vi "Update Shot Table.vi"(1 "Sort by AVG":bool, 2 "Site":string="ICE1", 3 "shotsArr":T1 {"Frag Rod" format="%.1f"; "UncorrectedAvgVel_PB" format="%.1f"; "UncorrectedRed_PB" format="%.1f"; "strikeVel_PB" format="%.1f"; "velLoss_PB" format="%.1f"; "avgVel_PB" format="%.1f"; "Redundant_Velocity" format="%.1f"; "Energy Loss (J)" format="%.3e"; "Projectile Mass" min=0 step=1 format="%.4f"; "Corrected residual" format="%.2f"; "Uncorrected Residual" format="%.1f"; "Corrected Impact" format="%.2f"; "Uncorrected Impact" format="%.1f"; "Shot Angle" max=90 step=1; "SHOT STATUS" items=["Partial", "Complete"]; "IMPACT VELOCITY" min=0 max=10000 step=0.1 format="%.1f"; "Barrel Temperature" format="%.1f"; "Powder Loading" format="%.4f"; "RESIDUAL  VELOCITY" min=0 max=10000 step=0.1 format="%.1f"}) -> (0 "shotTable OUT":string[][](array[string]))   [LabVIEW 2015]
uses:
  shotsArr.ctl
  Shot Record.ctl
panel:
  # "Chrono#1"
  # "Chrono#2"
  # "Average"
  # "Vel Loss"
  # "Strike Vel"
  # "Residual"
  # "Status"
  # "Depth"
  # "Diameter"
  # "Loading"
  # "Description"
  # "Order"
  # "Chrono#1"
  # "Chrono#2"
  # "Strike Vel"
  # "Status"
  # "Depth"
  # "Loading"
  # "Description"
  # "SPR"
  # "Order"
  # "Chrono#1"
  # "Chrono#2"
  # "Strike Vel"
  # "Status"
  # "Depth"
  # "Loading"
  # "Description"
  # "BRZ"
  # "Order"
  # "Corrected"
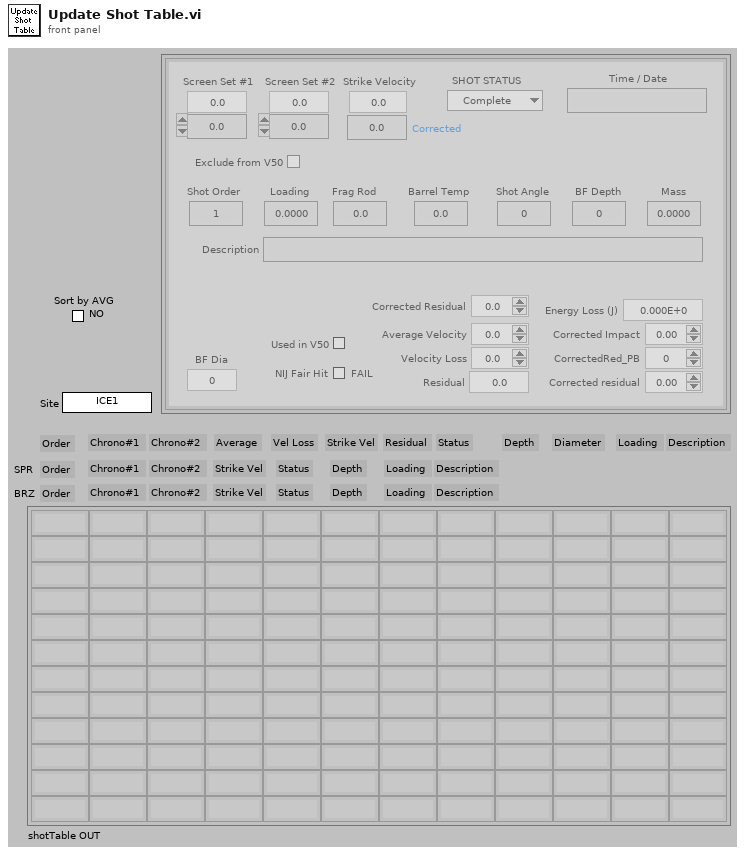
[diagram p1: front panel]
types:
  T1 = typedef "shotsArr.ctl" = T2[]
  T2 = typedef "Shot Record.ctl" = cluster{"Uncorrected Impact":sgl, "Uncorrected Residual":sgl, "avgVel_PB":sgl, "IMPACT VELOCITY":sgl, "RESIDUAL  VELOCITY ":sgl, "Shot Description":string, "Powder Loading ":sgl, "Barrel Temperature":sgl, "TIME / DATE":string, "shot order":i32, "SHOT STATUS":u16, "Shot Angle":u16, "Corrected Impact":sgl, "Corrected residual":sgl, "Projectile Mass":sgl, "usedv50":bool, "Energy Loss (J)":sgl, "BackFace\nDepth":sgl, "BackFace\nDiameter":sgl, "Redundant_Velocity":sgl, "velLoss_PB":sgl, "strikeVel_PB":sgl, "UncorrectedRed_PB":sgl, "CorrectedRed_PB":sgl, "UncorrectedAvgVel_PB":sgl, "V50userExcl":bool, "Frag Rod":sgl, "fairHit":bool}
  T3 = cluster{"[0]":string, "[1]":string, "[2]":string, "[3]":string, "[4]":string, "[5]":string, "[6]":string, "[7]":string, "[8]":string, "[9]":string, "[10]":string, "[11]":string}[]
  T4 = cluster{"[0]":string, "[1]":string, "[2]":string, "[3]":string, "[4]":string, "[5]":string, "[6]":string, "[7]":string, "[8]":string, "[9]":string, "[10]":string, "[11]":string}
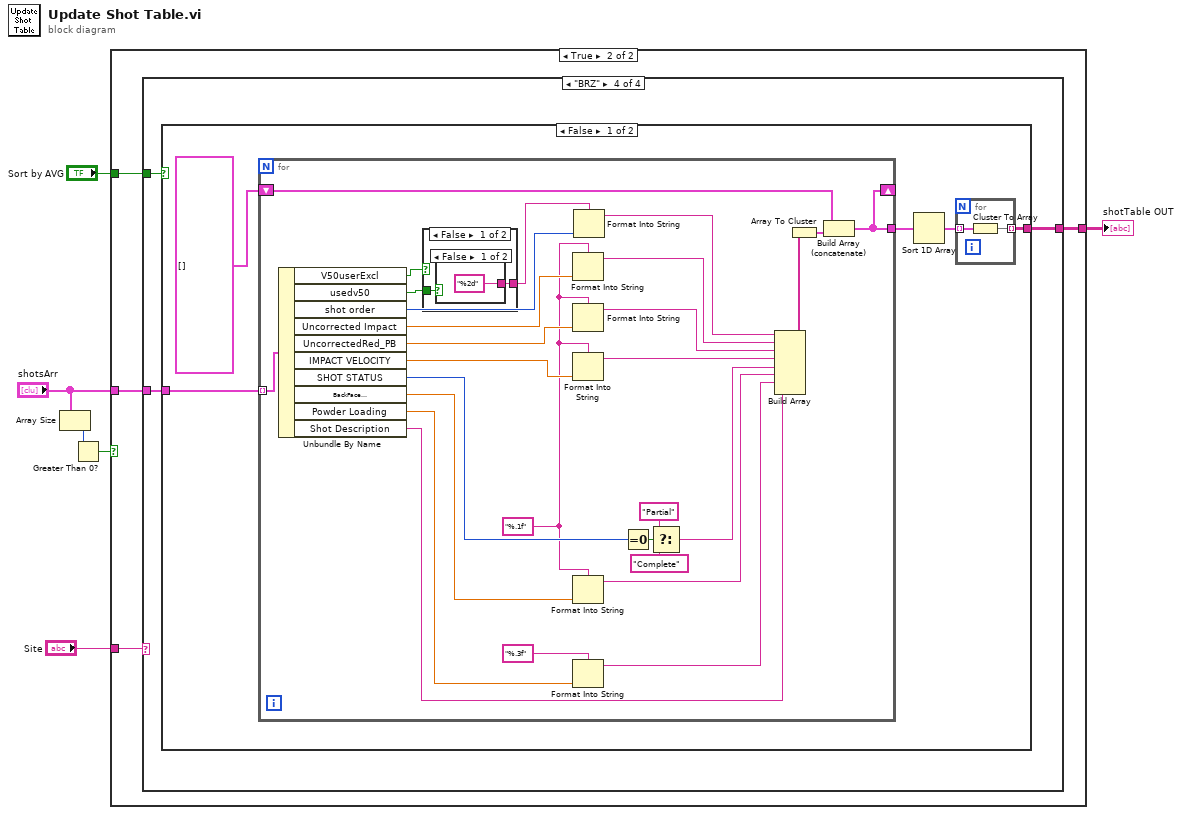
[diagram p0: block diagram]
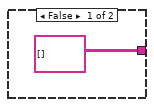
[diagram p2: hidden frame]
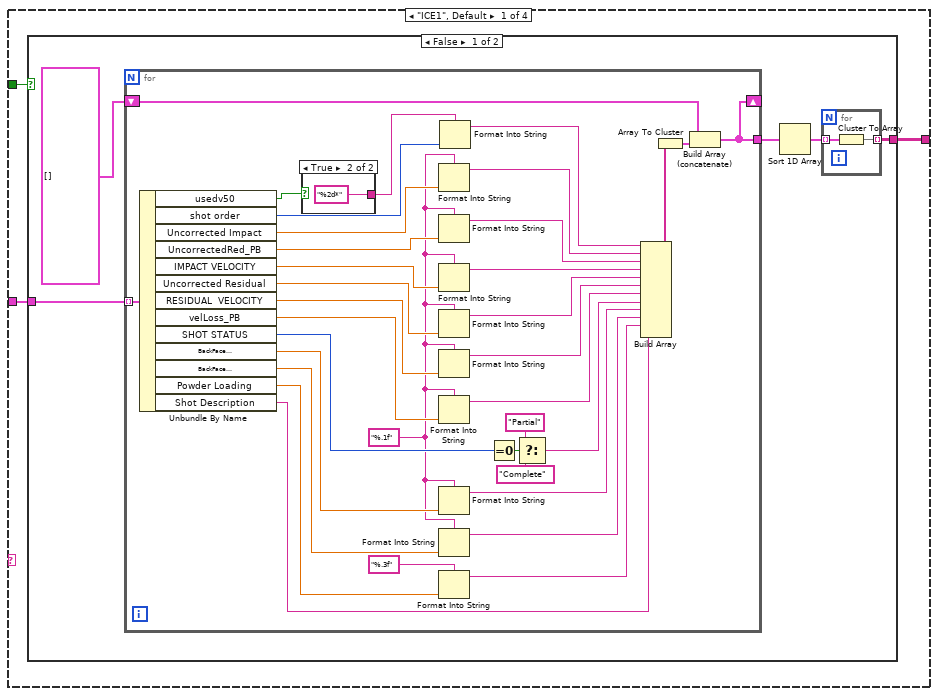
[diagram p3: hidden frame]
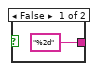
[diagram p4: hidden frame]
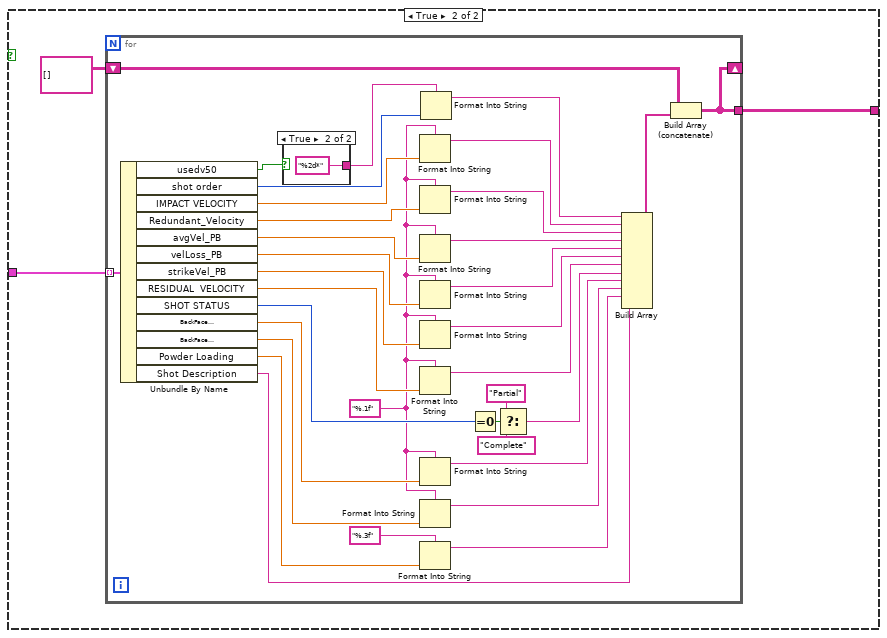
[diagram p5: hidden frame]
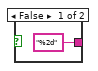
[diagram p6: hidden frame]
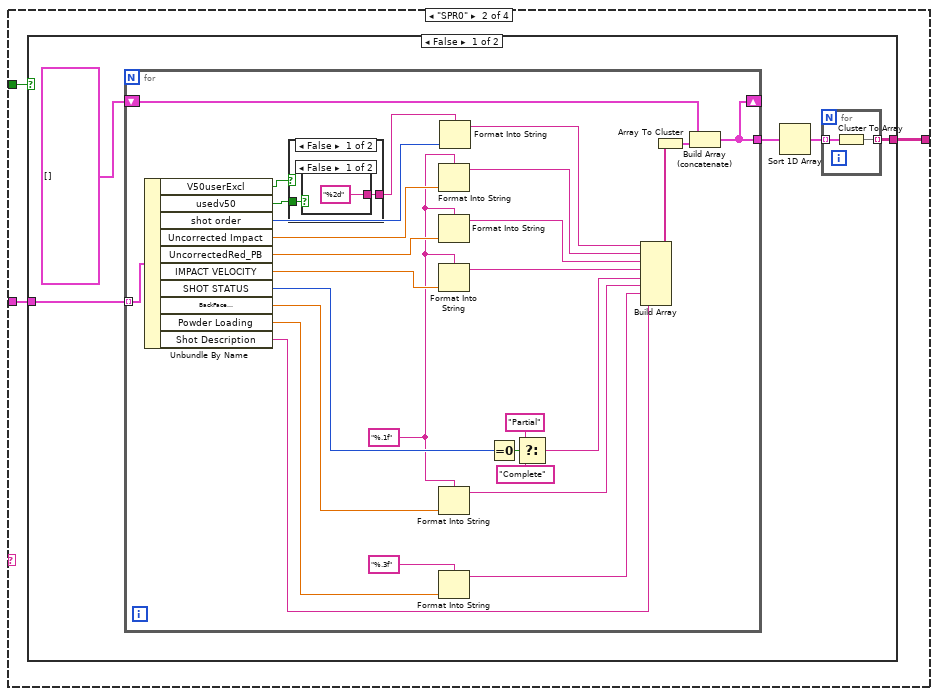
[diagram p7: hidden frame]
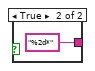
[diagram p8: hidden frame]
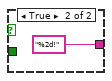
[diagram p9: hidden frame]
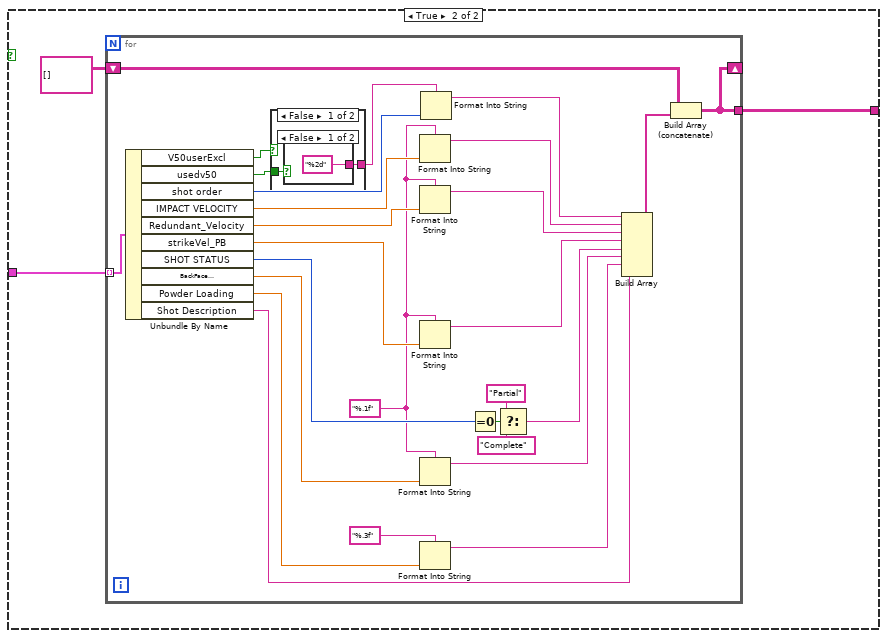
[diagram p10: hidden frame]
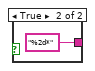
[diagram p11: hidden frame]
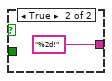
[diagram p12: hidden frame]
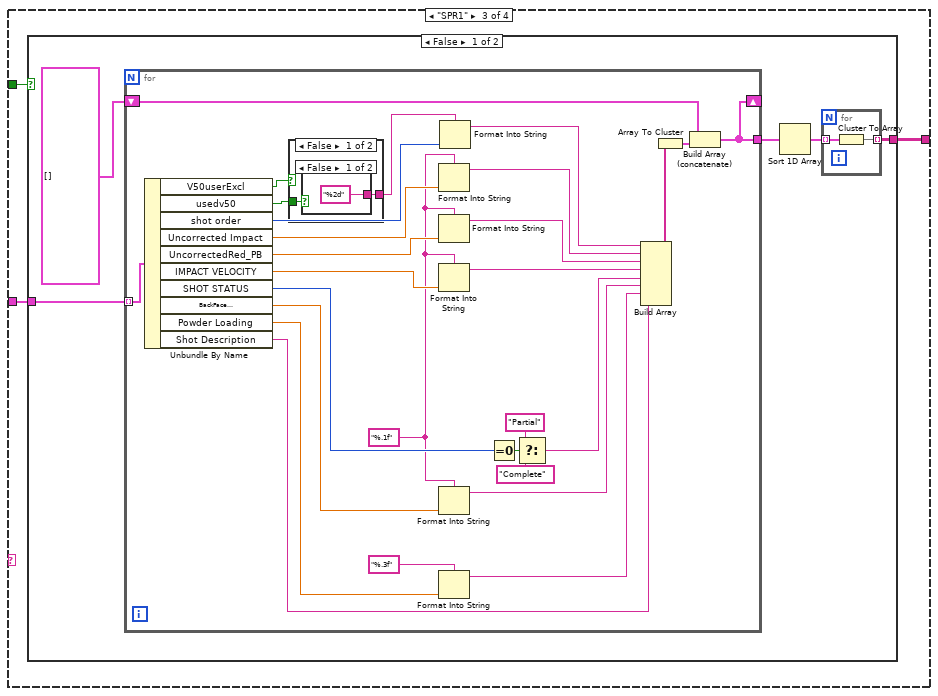
[diagram p13: hidden frame]
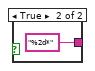
[diagram p14: hidden frame]
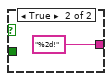
[diagram p15: hidden frame]
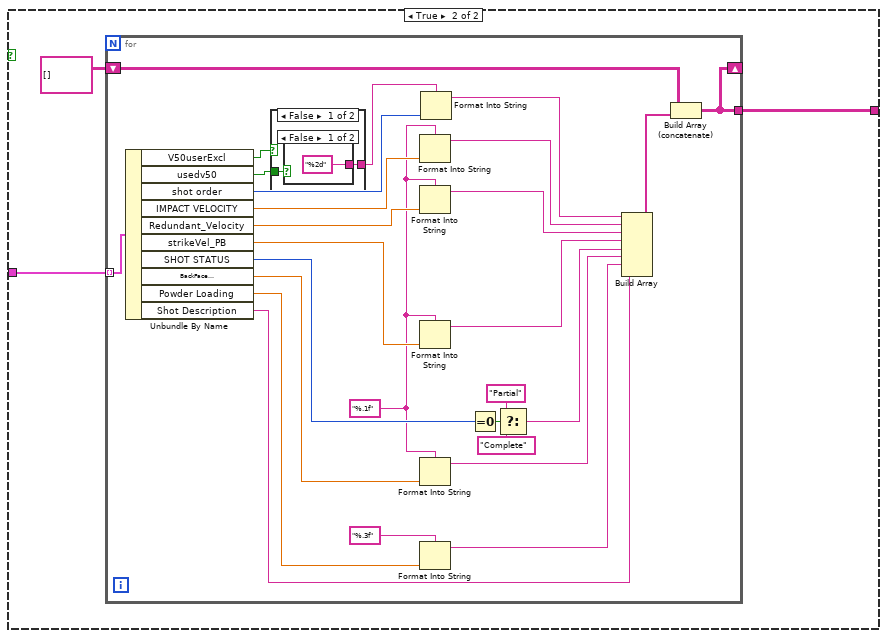
[diagram p16: hidden frame]
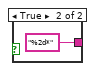
[diagram p17: hidden frame]
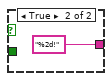
[diagram p18: hidden frame]
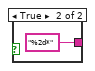
[diagram p19: hidden frame]
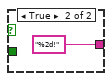
[diagram p20: hidden frame]
diagram:
  n1 = Array Size(array="shotsArr") -> (size(s)=w6:i32)
  n2 = Greater Than 0?(x=w6) -> (x > 0?=w4:bool)
  n3 = case shown="True" w4 {
    tunnel: "shotsArr" -> [_ w11]
    tunnel: [string[][] [] w10] -> w5
    tunnel: "Sort by AVG" -> [_ w9]
    tunnel: "Site" -> [_ w8]
    frame False {
    }
    frame True {
      n4 = case shown="\"BRZ\"" w8 {
        tunnel: w11 -> [w14 w100 w178 w256]
        tunnel: [w13 w99 w177 w255] -> w10
        tunnel: w9 -> [w12 w98 w176 w254]
        frame "ICE1", Default {
          n5 = case shown="False" w12 {
            tunnel: w14 -> [w19 w60]
            tunnel: [w17 w59] -> w13
            frame False {
              n6 = for {
                tunnel: w19 -> [w44] mode=indexing
                shift-right: [w52] -> _
                shift-left: T3 [] -> [w56]
                tunnel: [w52] -> w18
                w23 = "%.1f" ("Format String")
                n7 = Unbundle By Name(w44) -> ("usedv50"=w43:bool, "shot order"=w42:i32, "Uncorrected Impact"=w41:sgl, "UncorrectedRed_PB"=w40:sgl, "IMPACT VELOCITY"=w39:sgl, "Uncorrected Residual"=w38:sgl, "RESIDUAL  VELOCITY"=w37:sgl, "velLoss_PB"=w31:sgl, "SHOT STATUS"=w27:u16, "BackFace\nDepth"=w36:sgl, "BackFace\nDiameter"=w35:sgl, "Powder Loading"=w34:sgl, "Shot Description"=w33:string)
                n8 = case shown="True" w43 {
                  tunnel: ["%2d" "%2d*"] -> w51
                  frame False {
                  }
                  frame True {
                  }
                }
                n9 = Format Into String(format string=w23, w41) -> (resulting string=w53:string)  [unwired: 2 in, 1 out]
                n10 = Format Into String(format string=w23, w40) -> (resulting string=w54:string)  [unwired: 2 in, 1 out]
                n11 = Format Into String(format string=w23, w39) -> (resulting string=w32:string)  [unwired: 2 in, 1 out]
                n12 = Format Into String(format string=w23, w38) -> (resulting string=w49:string)  [unwired: 2 in, 1 out]
                n13 = Format Into String(format string=w23, w37) -> (resulting string=w48:string)  [unwired: 2 in, 1 out]
                n14 = Format Into String(format string=w23, w31) -> (resulting string=w25:string)  [unwired: 2 in, 1 out]
                n15 = Format Into String(format string=w23, w36) -> (resulting string=w47:string)  [unwired: 2 in, 1 out]
                n16 = Format Into String(format string=w23, w35) -> (resulting string=w46:string)  [unwired: 2 in, 1 out]
                n17 = Format Into String(format string="%.3f" ("Format String"), w34) -> (resulting string=w45:string)  [unwired: 2 in, 1 out]
                n18 = Format Into String(format string=w51, w42) -> (resulting string=w50:string)  [unwired: 2 in, 1 out]
                n19 = Equal To 0?(x=w27) -> (x = 0?=w28:bool)
                n20 = Select(t="Partial", s=w28, f="Complete") -> (s? t:f=w26:string)
                n21 = Build Array(w50, w53, w54, w32, w49, w48, w25, w26, w47, w46, w45, w33) -> (w55:string[])
                n22 = Array To Cluster(array=w55) -> (cluster=w22:T4)
                n23 = Build Array (concatenate)(w56, w22) -> (w52:T3)
              }
              n24 = Sort 1D Array(array=w18) -> (sorted array=w15:T3)
              n25 = for {
                tunnel: w15 -> [w21] mode=indexing
                tunnel: [w20] -> w17 mode=indexing
                n26 = Cluster To Array(cluster=w21) -> (array=w20:string[])
              }
            }
            frame True {
              n27 = for {
                tunnel: w60 -> [w84] mode=indexing
                shift-right: [w92] -> _
                shift-left: string[][] [] -> [w95]
                tunnel: [w92] -> w59
                w63 = "%.1f" ("Format String")
                n28 = Unbundle By Name(w84) -> ("usedv50"=w83:bool, "shot order"=w82:i32, "IMPACT VELOCITY"=w81:sgl, "Redundant_Velocity"=w80:sgl, "avgVel_PB"=w79:sgl, "velLoss_PB"=w78:sgl, "strikeVel_PB"=w77:sgl, "RESIDUAL  VELOCITY"=w71:sgl, "SHOT STATUS"=w67:u16, "BackFace\nDepth"=w76:sgl, "BackFace\nDiameter"=w75:sgl, "Powder Loading"=w74:sgl, "Shot Description"=w73:string)
                n29 = case shown="True" w83 {
                  tunnel: ["%2d" "%2d*"] -> w91
                  frame False {
                  }
                  frame True {
                  }
                }
                n30 = Format Into String(format string=w63, w81) -> (resulting string=w93:string)  [unwired: 2 in, 1 out]
                n31 = Format Into String(format string=w63, w80) -> (resulting string=w94:string)  [unwired: 2 in, 1 out]
                n32 = Format Into String(format string=w63, w79) -> (resulting string=w72:string)  [unwired: 2 in, 1 out]
                n33 = Format Into String(format string=w63, w78) -> (resulting string=w89:string)  [unwired: 2 in, 1 out]
                n34 = Format Into String(format string=w63, w77) -> (resulting string=w88:string)  [unwired: 2 in, 1 out]
                n35 = Format Into String(format string=w63, w71) -> (resulting string=w65:string)  [unwired: 2 in, 1 out]
                n36 = Format Into String(format string=w63, w76) -> (resulting string=w87:string)  [unwired: 2 in, 1 out]
                n37 = Format Into String(format string=w63, w75) -> (resulting string=w86:string)  [unwired: 2 in, 1 out]
                n38 = Format Into String(format string="%.3f" ("Format String"), w74) -> (resulting string=w85:string)  [unwired: 2 in, 1 out]
                n39 = Format Into String(format string=w91, w82) -> (resulting string=w90:string)  [unwired: 2 in, 1 out]
                n40 = Equal To 0?(x=w67) -> (x = 0?=w68:bool)
                n41 = Select(t="Partial", s=w68, f="Complete") -> (s? t:f=w66:string)
                n42 = Build Array(w90, w93, w94, w72, w89, w88, w65, w66, w87, w86, w85, w73) -> (w62:string[])
                n43 = Build Array (concatenate)(w95, w62) -> (w92:string[][])
              }
            }
          }
        }
        frame "SPR0" {
          n44 = case shown="False" w98 {
            tunnel: w100 -> [w105 w142]
            tunnel: [w103 w141] -> w99
            frame False {
              n45 = for {
                tunnel: w105 -> [w126] mode=indexing
                shift-right: [w131] -> _
                shift-left: T3 [] -> [w135]
                tunnel: [w131] -> w104
                w110 = "%.1f" ("Format String")
                n46 = Unbundle By Name(w126) -> ("V50userExcl"=w108:bool, "usedv50"=w125:bool, "shot order"=w124:i32, "Uncorrected Impact"=w123:sgl, "UncorrectedRed_PB"=w122:sgl, "IMPACT VELOCITY"=w121:sgl, "SHOT STATUS"=w113:u16, "BackFace\nDepth"=w120:sgl, "Powder Loading"=w119:sgl, "Shot Description"=w118:string)
                n47 = case shown="False" w108 {
                  tunnel: [w137 "%2d!"] -> w130
                  tunnel: w125 -> [w136 _]
                  frame False {
                    n48 = case shown="False" w136 {
                      tunnel: ["%2d" "%2d*"] -> w137
                      frame False {
                      }
                      frame True {
                      }
                    }
                  }
                  frame True {
                  }
                }
                n49 = Format Into String(format string=w110, w123) -> (resulting string=w132:string)  [unwired: 2 in, 1 out]
                n50 = Format Into String(format string=w110, w122) -> (resulting string=w133:string)  [unwired: 2 in, 1 out]
                n51 = Format Into String(format string=w110, w121) -> (resulting string=w117:string)  [unwired: 2 in, 1 out]
                n52 = Format Into String(format string=w110, w120) -> (resulting string=w128:string)  [unwired: 2 in, 1 out]
                n53 = Format Into String(format string="%.3f" ("Format String"), w119) -> (resulting string=w127:string)  [unwired: 2 in, 1 out]
                n54 = Format Into String(format string=w130, w124) -> (resulting string=w129:string)  [unwired: 2 in, 1 out]
                n55 = Equal To 0?(x=w113) -> (x = 0?=w114:bool)
                n56 = Select(t="Partial", s=w114, f="Complete") -> (s? t:f=w112:string)
                n57 = Build Array(w129, w132, w133, w117, w112, w128, w127, w118) -> (w134:string[])
                n58 = Array To Cluster(array=w134) -> (cluster=w109:T4)
                n59 = Build Array (concatenate)(w135, w109) -> (w131:T3)
              }
              n60 = Sort 1D Array(array=w104) -> (sorted array=w101:T3)
              n61 = for {
                tunnel: w101 -> [w107] mode=indexing
                tunnel: [w106] -> w103 mode=indexing
                n62 = Cluster To Array(cluster=w107) -> (array=w106:string[])
              }
            }
            frame True {
              n63 = for {
                tunnel: w142 -> [w162] mode=indexing
                shift-right: [w167] -> _
                shift-left: string[][] [] -> [w170]
                tunnel: [w167] -> w141
                w148 = "%.1f" ("Format String")
                n64 = Unbundle By Name(w162) -> ("V50userExcl"=w145:bool, "usedv50"=w146:bool, "shot order"=w161:i32, "IMPACT VELOCITY"=w160:sgl, "Redundant_Velocity"=w159:sgl, "strikeVel_PB"=w158:sgl, "SHOT STATUS"=w151:u16, "BackFace\nDepth"=w157:sgl, "Powder Loading"=w156:sgl, "Shot Description"=w155:string)
                n65 = case shown="False" w145 {
                  tunnel: [w172 "%2d!"] -> w144
                  tunnel: w146 -> [w171 _]
                  frame False {
                    n66 = case shown="False" w171 {
                      tunnel: ["%2d" "%2d*"] -> w172
                      frame False {
                      }
                      frame True {
                      }
                    }
                  }
                  frame True {
                  }
                }
                n67 = Format Into String(format string=w148, w160) -> (resulting string=w168:string)  [unwired: 2 in, 1 out]
                n68 = Format Into String(format string=w148, w159) -> (resulting string=w169:string)  [unwired: 2 in, 1 out]
                n69 = Format Into String(format string=w148, w158) -> (resulting string=w165:string)  [unwired: 2 in, 1 out]
                n70 = Format Into String(format string=w148, w157) -> (resulting string=w164:string)  [unwired: 2 in, 1 out]
                n71 = Format Into String(format string="%.3f" ("Format String"), w156) -> (resulting string=w163:string)  [unwired: 2 in, 1 out]
                n72 = Format Into String(format string=w144, w161) -> (resulting string=w166:string)  [unwired: 2 in, 1 out]
                n73 = Equal To 0?(x=w151) -> (x = 0?=w152:bool)
                n74 = Select(t="Partial", s=w152, f="Complete") -> (s? t:f=w150:string)
                n75 = Build Array(w166, w168, w169, w165, w150, w164, w163, w155) -> (w147:string[])
                n76 = Build Array (concatenate)(w170, w147) -> (w167:string[][])
              }
            }
          }
        }
        frame "SPR1" {
          n77 = case shown="False" w176 {
            tunnel: w178 -> [w183 w220]
            tunnel: [w181 w219] -> w177
            frame False {
              n78 = for {
                tunnel: w183 -> [w204] mode=indexing
                shift-right: [w209] -> _
                shift-left: T3 [] -> [w213]
                tunnel: [w209] -> w182
                w188 = "%.1f" ("Format String")
                n79 = Unbundle By Name(w204) -> ("V50userExcl"=w186:bool, "usedv50"=w203:bool, "shot order"=w202:i32, "Uncorrected Impact"=w201:sgl, "UncorrectedRed_PB"=w200:sgl, "IMPACT VELOCITY"=w199:sgl, "SHOT STATUS"=w191:u16, "BackFace\nDepth"=w198:sgl, "Powder Loading"=w197:sgl, "Shot Description"=w196:string)
                n80 = case shown="False" w186 {
                  tunnel: [w215 "%2d!"] -> w208
                  tunnel: w203 -> [w214 _]
                  frame False {
                    n81 = case shown="False" w214 {
                      tunnel: ["%2d" "%2d*"] -> w215
                      frame False {
                      }
                      frame True {
                      }
                    }
                  }
                  frame True {
                  }
                }
                n82 = Format Into String(format string=w188, w201) -> (resulting string=w210:string)  [unwired: 2 in, 1 out]
                n83 = Format Into String(format string=w188, w200) -> (resulting string=w211:string)  [unwired: 2 in, 1 out]
                n84 = Format Into String(format string=w188, w199) -> (resulting string=w195:string)  [unwired: 2 in, 1 out]
                n85 = Format Into String(format string=w188, w198) -> (resulting string=w206:string)  [unwired: 2 in, 1 out]
                n86 = Format Into String(format string="%.3f" ("Format String"), w197) -> (resulting string=w205:string)  [unwired: 2 in, 1 out]
                n87 = Format Into String(format string=w208, w202) -> (resulting string=w207:string)  [unwired: 2 in, 1 out]
                n88 = Equal To 0?(x=w191) -> (x = 0?=w192:bool)
                n89 = Select(t="Partial", s=w192, f="Complete") -> (s? t:f=w190:string)
                n90 = Build Array(w207, w210, w211, w195, w190, w206, w205, w196) -> (w212:string[])
                n91 = Array To Cluster(array=w212) -> (cluster=w187:T4)
                n92 = Build Array (concatenate)(w213, w187) -> (w209:T3)
              }
              n93 = Sort 1D Array(array=w182) -> (sorted array=w179:T3)
              n94 = for {
                tunnel: w179 -> [w185] mode=indexing
                tunnel: [w184] -> w181 mode=indexing
                n95 = Cluster To Array(cluster=w185) -> (array=w184:string[])
              }
            }
            frame True {
              n96 = for {
                tunnel: w220 -> [w240] mode=indexing
                shift-right: [w245] -> _
                shift-left: string[][] [] -> [w248]
                tunnel: [w245] -> w219
                w226 = "%.1f" ("Format String")
                n97 = Unbundle By Name(w240) -> ("V50userExcl"=w223:bool, "usedv50"=w224:bool, "shot order"=w239:i32, "IMPACT VELOCITY"=w238:sgl, "Redundant_Velocity"=w237:sgl, "strikeVel_PB"=w236:sgl, "SHOT STATUS"=w229:u16, "BackFace\nDepth"=w235:sgl, "Powder Loading"=w234:sgl, "Shot Description"=w233:string)
                n98 = case shown="False" w223 {
                  tunnel: [w250 "%2d!"] -> w222
                  tunnel: w224 -> [w249 _]
                  frame False {
                    n99 = case shown="False" w249 {
                      tunnel: ["%2d" "%2d*"] -> w250
                      frame False {
                      }
                      frame True {
                      }
                    }
                  }
                  frame True {
                  }
                }
                n100 = Format Into String(format string=w226, w238) -> (resulting string=w246:string)  [unwired: 2 in, 1 out]
                n101 = Format Into String(format string=w226, w237) -> (resulting string=w247:string)  [unwired: 2 in, 1 out]
                n102 = Format Into String(format string=w226, w236) -> (resulting string=w243:string)  [unwired: 2 in, 1 out]
                n103 = Format Into String(format string=w226, w235) -> (resulting string=w242:string)  [unwired: 2 in, 1 out]
                n104 = Format Into String(format string="%.3f" ("Format String"), w234) -> (resulting string=w241:string)  [unwired: 2 in, 1 out]
                n105 = Format Into String(format string=w222, w239) -> (resulting string=w244:string)  [unwired: 2 in, 1 out]
                n106 = Equal To 0?(x=w229) -> (x = 0?=w230:bool)
                n107 = Select(t="Partial", s=w230, f="Complete") -> (s? t:f=w228:string)
                n108 = Build Array(w244, w246, w247, w243, w228, w242, w241, w233) -> (w225:string[])
                n109 = Build Array (concatenate)(w248, w225) -> (w245:string[][])
              }
            }
          }
        }
        frame "BRZ" {
          n110 = case shown="False" w254 {
            tunnel: w256 -> [w261 w298]
            tunnel: [w259 w297] -> w255
            frame False {
              n111 = for {
                tunnel: w261 -> [w282] mode=indexing
                shift-right: [w287] -> _
                shift-left: T3 [] -> [w291]
                tunnel: [w287] -> w260
                w266 = "%.1f" ("Format String")
                n112 = Unbundle By Name(w282) -> ("V50userExcl"=w264:bool, "usedv50"=w281:bool, "shot order"=w280:i32, "Uncorrected Impact"=w279:sgl, "UncorrectedRed_PB"=w278:sgl, "IMPACT VELOCITY"=w277:sgl, "SHOT STATUS"=w269:u16, "BackFace\nDepth"=w276:sgl, "Powder Loading"=w275:sgl, "Shot Description"=w274:string)
                n113 = case shown="False" w264 {
                  tunnel: [w293 "%2d!"] -> w286
                  tunnel: w281 -> [w292 _]
                  frame False {
                    n114 = case shown="False" w292 {
                      tunnel: ["%2d" "%2d*"] -> w293
                      frame False {
                      }
                      frame True {
                      }
                    }
                  }
                  frame True {
                  }
                }
                n115 = Format Into String(format string=w266, w279) -> (resulting string=w288:string)  [unwired: 2 in, 1 out]
                n116 = Format Into String(format string=w266, w278) -> (resulting string=w289:string)  [unwired: 2 in, 1 out]
                n117 = Format Into String(format string=w266, w277) -> (resulting string=w273:string)  [unwired: 2 in, 1 out]
                n118 = Format Into String(format string=w266, w276) -> (resulting string=w284:string)  [unwired: 2 in, 1 out]
                n119 = Format Into String(format string="%.3f" ("Format String"), w275) -> (resulting string=w283:string)  [unwired: 2 in, 1 out]
                n120 = Format Into String(format string=w286, w280) -> (resulting string=w285:string)  [unwired: 2 in, 1 out]
                n121 = Equal To 0?(x=w269) -> (x = 0?=w270:bool)
                n122 = Select(t="Partial", s=w270, f="Complete") -> (s? t:f=w268:string)
                n123 = Build Array(w285, w288, w289, w273, w268, w284, w283, w274) -> (w290:string[])
                n124 = Array To Cluster(array=w290) -> (cluster=w265:T4)
                n125 = Build Array (concatenate)(w291, w265) -> (w287:T3)
              }
              n126 = Sort 1D Array(array=w260) -> (sorted array=w257:T3)
              n127 = for {
                tunnel: w257 -> [w263] mode=indexing
                tunnel: [w262] -> w259 mode=indexing
                n128 = Cluster To Array(cluster=w263) -> (array=w262:string[])
              }
            }
            frame True {
              n129 = for {
                tunnel: w298 -> [w318] mode=indexing
                shift-right: [w323] -> _
                shift-left: string[][] [] -> [w326]
                tunnel: [w323] -> w297
                w304 = "%.1f" ("Format String")
                n130 = Unbundle By Name(w318) -> ("V50userExcl"=w301:bool, "usedv50"=w302:bool, "shot order"=w317:i32, "IMPACT VELOCITY"=w316:sgl, "Redundant_Velocity"=w315:sgl, "strikeVel_PB"=w314:sgl, "SHOT STATUS"=w307:u16, "BackFace\nDepth"=w313:sgl, "Powder Loading"=w312:sgl, "Shot Description"=w311:string)
                n131 = case shown="False" w301 {
                  tunnel: [w328 "%2d!"] -> w300
                  tunnel: w302 -> [w327 _]
                  frame False {
                    n132 = case shown="False" w327 {
                      tunnel: ["%2d" "%2d*"] -> w328
                      frame False {
                      }
                      frame True {
                      }
                    }
                  }
                  frame True {
                  }
                }
                n133 = Format Into String(format string=w304, w316) -> (resulting string=w324:string)  [unwired: 2 in, 1 out]
                n134 = Format Into String(format string=w304, w315) -> (resulting string=w325:string)  [unwired: 2 in, 1 out]
                n135 = Format Into String(format string=w304, w314) -> (resulting string=w321:string)  [unwired: 2 in, 1 out]
                n136 = Format Into String(format string=w304, w313) -> (resulting string=w320:string)  [unwired: 2 in, 1 out]
                n137 = Format Into String(format string="%.3f" ("Format String"), w312) -> (resulting string=w319:string)  [unwired: 2 in, 1 out]
                n138 = Format Into String(format string=w300, w317) -> (resulting string=w322:string)  [unwired: 2 in, 1 out]
                n139 = Equal To 0?(x=w307) -> (x = 0?=w308:bool)
                n140 = Select(t="Partial", s=w308, f="Complete") -> (s? t:f=w306:string)
                n141 = Build Array(w322, w324, w325, w321, w306, w320, w319, w311) -> (w303:string[])
                n142 = Build Array (concatenate)(w326, w303) -> (w323:string[][])
              }
            }
          }
        }
      }
    }
  }
  "shotTable OUT" <- w5
